vi "Set ClockID T0.vi"(8 "error in (no error)":errorcluster, 11 "CIFCorePlugin in":refnum<class "CIFCorePlugin.lvclass">) -> (0 "error out":errorcluster, 3 "CIFCorePlugin out":refnum<class "CIFCorePlugin.lvclass">)   [LabVIEW 2021, in "CIFCorePlugin.lvclass"]
uses:
  CIFCorePlugin.lvclass
  CIFCorePlugin.lvclass/CIFCorePlugin.ctl
  <vilib>/CIF Foundation/CIF Utilities/Time/SubVIs/Add Error.vi
  <vilib>/CIF Foundation/CIF Utilities/Errors/Append Error Location.vi
  <vilib>/CIF Foundation/CIF Utilities/Time/Time_CIF_U.lvlib
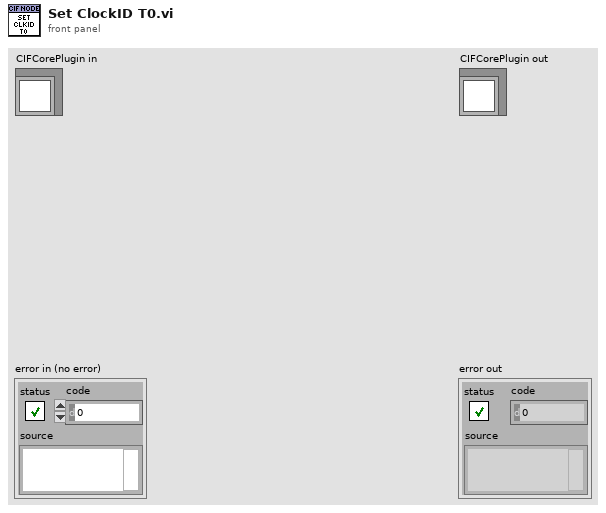
[diagram p1: front panel]
types:
  T1 = typedef "Time_CIF_U.lvlib/Clock Conversion Map.ctl" = map{u8, cluster{"Last Reset":i64, "Offset Pair":T2, "Slope":dbl, "1/Slope":dbl}}
  T2 = typedef "Time_CIF_U.lvlib/Timestamp Pair.ctl" = cluster{"System Time":i64, "External Time":i64}
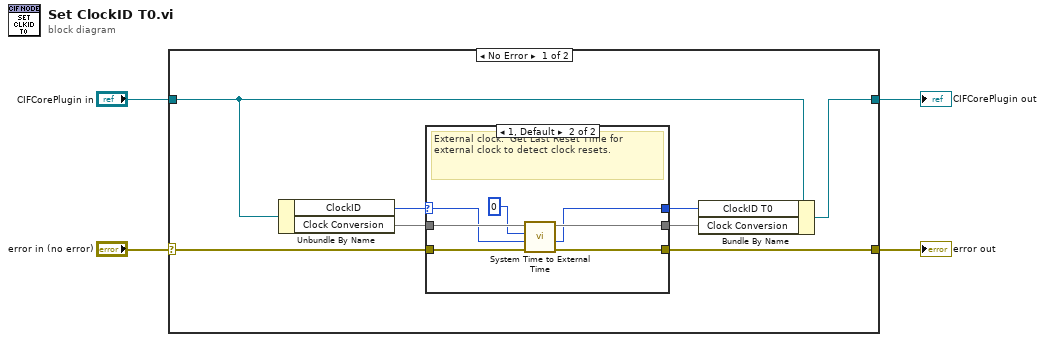
[diagram p0: block diagram]
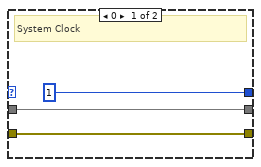
[diagram p2: hidden frame]
diagram:
  n1 = case shown="No Error" "error in (no error)" {
    selector: "error in (no error)" -> [w11 w24]
    tunnel: [w5 w24] -> w1
    tunnel: [w7 w23] -> w2
    tunnel: "CIFCorePlugin in" -> [w10 w23]
    frame No Error {
      n2 = Unbundle By Name(w10) -> ("ClockID"=w6:u8, "Clock Conversion"=w12:T1)
      n3 = case shown="1, Default" w6 {
        selector: w6 -> [_ w17]
        tunnel: w12 -> [w13 w22]
        tunnel: w11 -> [w15 w20]
        tunnel: [w15 w19] -> w5
        tunnel: [w13 w21] -> w9
        tunnel: [i64 1 ("Last Reset Time") w18] -> w8
        frame 0 {
          # "System Clock"
        }
        frame 1, Default {
          # "External clock.  Get Last Reset Time for external clock to detect clock resets."
          n4 = call <vilib>:"System Time to External Time.vi"("error in (no error)"=w20, "ClockID"=w17, "System Time"=i64 0, "Clock Convert Map in"=w22) -> ("error out"=w19:errorcluster, "Last Reset Time"=w18:i64, "Clock Convert Map out"=w21:T1)  [unwired: 4 in, 1 out]
        }
      }
      n5 = Bundle By Name(cluster=w10, "ClockID T0"=w8, "Clock Conversion"=w9) -> (w7:refnum<class "CIFCorePlugin.lvclass">)
    }
    frame Error {
    }
  }
  "error out" <- w1
  "CIFCorePlugin out" <- w2
